vi "AIT 15533 - Add Multiple Channels.vi"(8 "error in (no error)":errorcluster, 11 "Node Ptr":u64 format="%.0x") -> (0 "error out":errorcluster)   [LabVIEW 2013, in "AIT 1553 Custom Device.lvlib"]
uses:
  AIT 1553 Custom Device.lvlib
  Controls/Channel Setup.ctl
  <vilib>/NI Veristand/Custom Device API/Custom Device Channel Type.ctl
  <vilib>/NI Veristand/Custom Device API/Custom Device Channel.ctl
  Controls and Global/Global.vi
  <vilib>/NI Veristand/Custom Device API/Get Item Property (U32 Array).vi
  <vilib>/NI Veristand/Custom Device API/Get Item Property (Boolean).vi
  <vilib>/NI Veristand/Custom Device API/Custom Device API.lvlib
panel:
  in  "Cancel":bool
  in  "OK":bool
  in  "Parameters to Add":T1[](array[typedef]) {"Scale Offset" format="%.2f"; "Scale Factor" format="%.2f"; "Number of Bits" min=1 max=32 step=1; "Start Bit" min=0 max=31 step=1; "Start Word" min=1 max=31 step=1}
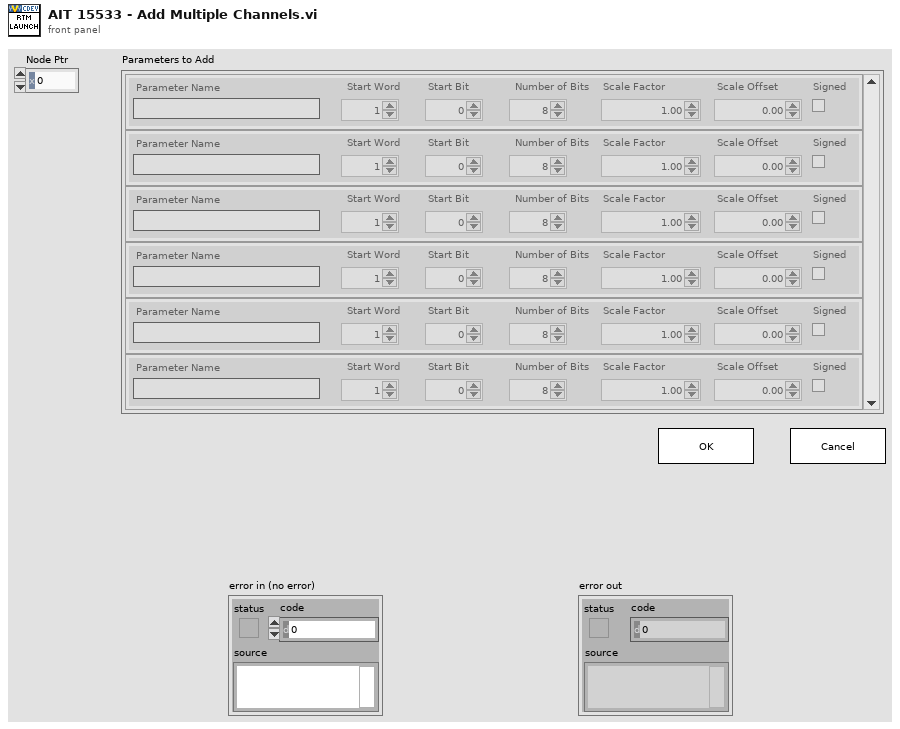
[diagram p1: front panel]
types:
  T1 = typedef "AIT 1553 Custom Device.lvlib/Channel Setup.ctl" = cluster{"Parameter Name":string, "Start Word":i32, "Start Bit":i32, "Number of Bits":i32, "Scale Factor":dbl, "Scale Offset":dbl, "Signed":bool}
  T2 = typedef "Custom Device API.lvlib/Custom Device Channel Type.ctl" = enum16{"Input", "Output"}
  T3 = typedef "Custom Device API.lvlib/Custom Device Channel.ctl" = cluster{"Type":T2, "Units":string, "Default Value":dbl, "Faultable":bool, "Scalable":bool}
  T4 = typedef "Custom Device API.lvlib/Custom Device Item Ref.ctl" = u64
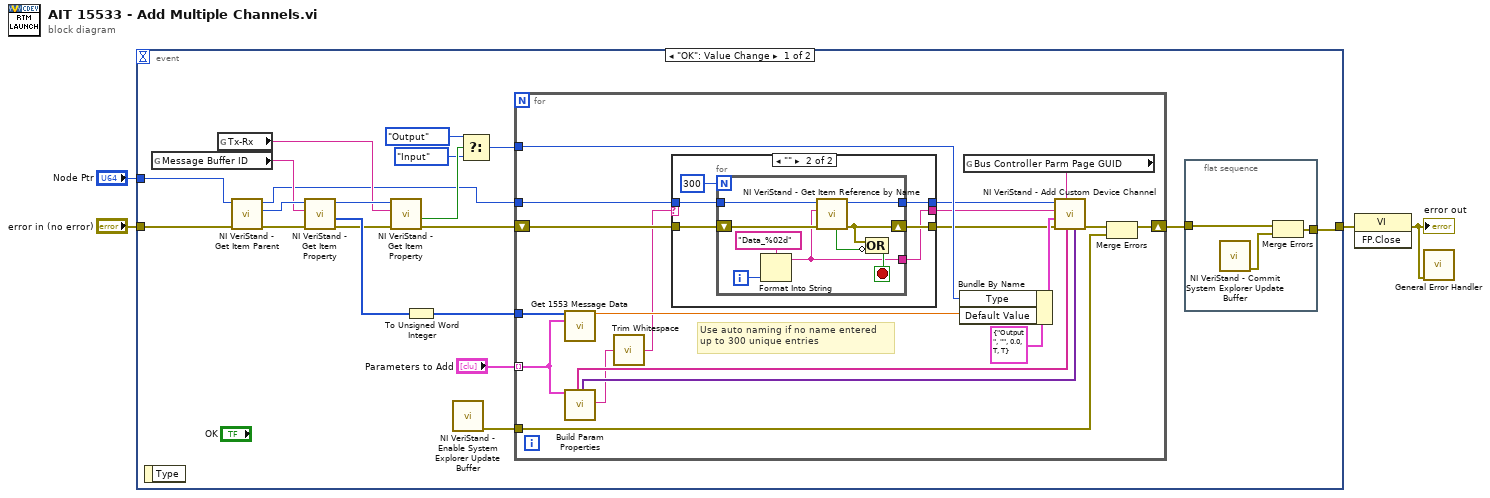
[diagram p0: block diagram]
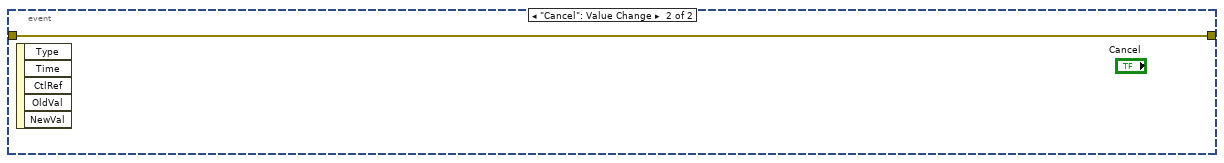
[diagram p3: hidden frame]
diagram:
  n1 = event shown="[0] \"OK\": Value Change" {
    selector: _ -> [_ _]
    dyn-events: _ -> [_ _]
    timeout: _ -> [_ _]
    tunnel: [w24 w65] -> w2
    tunnel: "error in (no error)" -> [w9 w65]
    tunnel: "Node Ptr" -> [w10 _]
    event "OK": Value Change {
      n2 = event-data() -> ()  [unwired: 1 in, 1 out]
      n3 = global read "Global.vi" "Message Buffer ID"() -> (w21:string)
      n4 = global read "Global.vi" "Tx-Rx"() -> (w16:string)
      n5 = call <vilib>:"NI VeriStand - Get Item Parent.vi"("error in (no error)"=w9, "Item Ref in"=w10) -> ("error out"=w22:errorcluster, "Parent Ref"=w23:T4, "Item Ref out"=w6:T4)  [unwired: 6 in, 1 out]
      n6 = call-poly <vilib>:"NI VeriStand - Get Item Property.vi"("error in (no error)"=w22, "Property Name"=w21, "Item Ref in"=w23) -> ("error out"=w18:errorcluster, "Value"=w20:u32[], "Item Ref out"=w17:T4)  [unwired: 5 in, 1 out]
      n7 = call-poly <vilib>:"NI VeriStand - Get Item Property.vi"("error in (no error)"=w18, "Property Name"=w16, "Item Ref in"=w17) -> ("error out"=w11:errorcluster, "Value"=w15:bool)  [unwired: 5 in, 2 out]
      n8 = To Unsigned Word Integer(number=w20) -> (unsigned 16bit integer=w19:u16[])
      n9 = call <vilib>:"NI VeriStand - Enable System Explorer Update Buffer.vi"() -> ("error out"=w8:errorcluster)  [unwired: 11 in]
      n10 = Select(t=Custom_Device_Channel_Type."Output" ("Type"), s=w15, f=Custom_Device_Channel_Type."Input" ("Type")) -> (s? t:f=w12:T2)
      n11 = for {
        tunnel: w19 -> [w40]
        tunnel: w12 -> [w37]
        tunnel: w6 -> [w32]
        tunnel: w8 -> [w26]
        tunnel: "Parameters to Add" -> [w31] mode=indexing
        shift-right: [w25] -> w5
        shift-left: w11 -> [w35]
        # "Use auto naming if no name entered\nup to 300 unique entries"
        n12 = call "Get 1553 Message Data.vi"("MSG DATA"=w40, "1553 Parameter"=w31) -> ("Value"=w39:dbl)  [unwired: 12 in, 1 out]
        n13 = call "Build Param Properties.vi"("1553 Parameter"=w31) -> ("Prop Names"=w42:string[], "Prop Values"=w41:variant[], "name"=w30:string)  [unwired: 10 in, 6 out]
        n14 = call <vilib>:"Trim Whitespace.vi"("string"=w30) -> ("trimmed string"=w28:string)  [unwired: 1 in]
        n15 = case shown="\"\"" w28 {
          selector: w28 -> [w46 _]
          tunnel: w35 -> [w44 w52]
          tunnel: [w44 w51] -> w34
          tunnel: [w45 w50] -> w33
          tunnel: w32 -> [w45 w48]
          tunnel: [w46 w47] -> w29
          frame Default {
            # "Valid Name String Entered"
          }
          frame "" {
            n16 = for {
              N: 300 -> [_]
              tunnel: w48 -> [w61]
              tunnel: [w56] -> w50
              tunnel: [w53] -> w47
              shift-right: [w58] -> w51
              shift-left: w52 -> [w60]
              i -> [w55]
              stop <- w59 stop-if-true
              n17 = Format Into String(format string="Data_%02d" ("name"), w55) -> (resulting string=w53:string)  [unwired: 2 in, 1 out]
              n18 = call <vilib>:"NI VeriStand - Get Item Reference by Name.vi"("error in (no error)"=w60, "Item Name"=w53, "Parent Ref in"=w61) -> ("error out"=w58:errorcluster, "Parent Ref out"=w56:T4, "Found"=w57:bool)  [unwired: 5 in, 1 out]
              n19 = Compound Arithmetic op=OR(w58, invert w57) -> (w59:bool)
            }
          }
        }
        n20 = Bundle By Name(cluster=T3 {"Type"=enum."Output", "Units"="", "Default Value"=0.0, "Faultable"=TRUE, "Scalable"=TRUE} ("Channel"), "Type"=w37, "Default Value"=w39) -> (w36:T3)
        n21 = global read "Global.vi" "Bus Controller Parm Page GUID"() -> (w43:string)
        n22 = call <vilib>:"NI VeriStand - Add Custom Device Channel.vi"("Property Values"=w41, "Property names"=w42, "GUID (Default Channel)"=w43, "error in (no error)"=w34, "Channel"=w36, "Channel Name"=w29, "Parent Ref in"=w33) -> ("error out"=w27:errorcluster)  [unwired: 1 in, 3 out]
        n23 = Merge Errors(w27, w26) -> (w25:errorcluster)
      }
      n24 = flat-sequence {
        tunnel: w5 -> [w64]
        tunnel: [w62] -> w24
        frame #0 {
          n25 = call <vilib>:"NI VeriStand - Commit System Explorer Update Buffer.vi"() -> ("error out"=w63:errorcluster)  [unwired: 11 in]
          n26 = Merge Errors(w64, w63) -> (w62:errorcluster)
        }
      }
    }
    event "Cancel": Value Change {
      n27 = event-data() -> ()  [unwired: 1 in, 5 out]
    }
  }
  n28 = invoke class="VI" method="FP.Close"(error in=w2) -> (error out=w1:errorcluster)  [unwired: 2 in, 2 out]
  "error out" <- w1
  n29 = call <vilib>:"General Error Handler.vi"("error in (no error)"=w1) -> ()  [unwired: 10 in, 5 out]
